vi "Write Unique Test ID.vi"(10 "Unique Test ID":string, 11 "Test Assert in":refnum<class "Test Assert.lvclass">) -> (3 "Test Assert out":refnum<class "Test Assert.lvclass">)   [LabVIEW 2013, in "Caraya.lvlib" / "Test Assert.lvclass"]
uses:
  Test Assert.lvclass
  Test Assert.lvclass/Test Assert.ctl
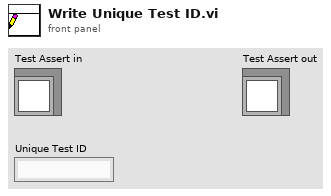
[diagram p1: front panel]
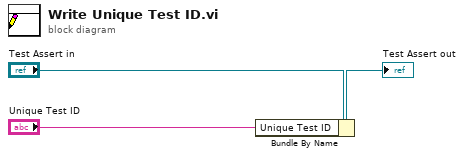
[diagram p0: block diagram]
diagram:
  n1 = Bundle By Name(cluster="Test Assert in", "Unique Test ID"="Unique Test ID") -> (→"Test Assert out":refnum<class "Test Assert.lvclass">)
